vi "trapezoidal.vi"(5 "offset":dbl, 6 "sampling info":cluster{"Fs":dbl, "#s":dbl}={"Fs"=1000.0, "#s"=1000.0} {"Fs" format="%.2p"}, 9 "phase":dbl, 10 "amplitude":dbl, 11 "frequency":i32) -> (2 "signal":waveform(dbl)(graph))   [LabVIEW 2019]
uses:
  <vilib>/Analysis/1siggen.llb/Ramp Pattern by Samples.vi
  <vilib>/Analysis/NI_AALBase.lvlib
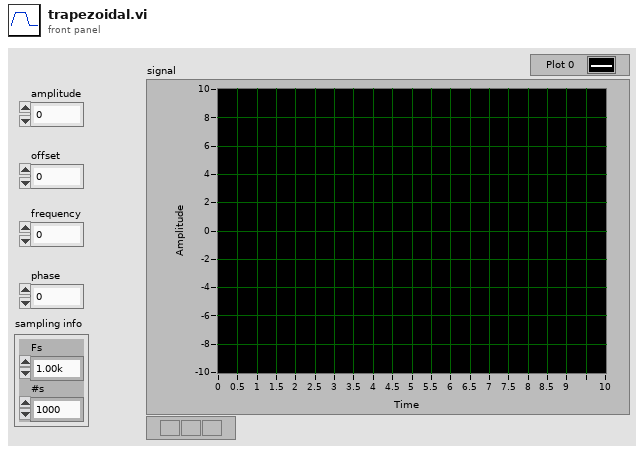
[diagram p1: front panel]
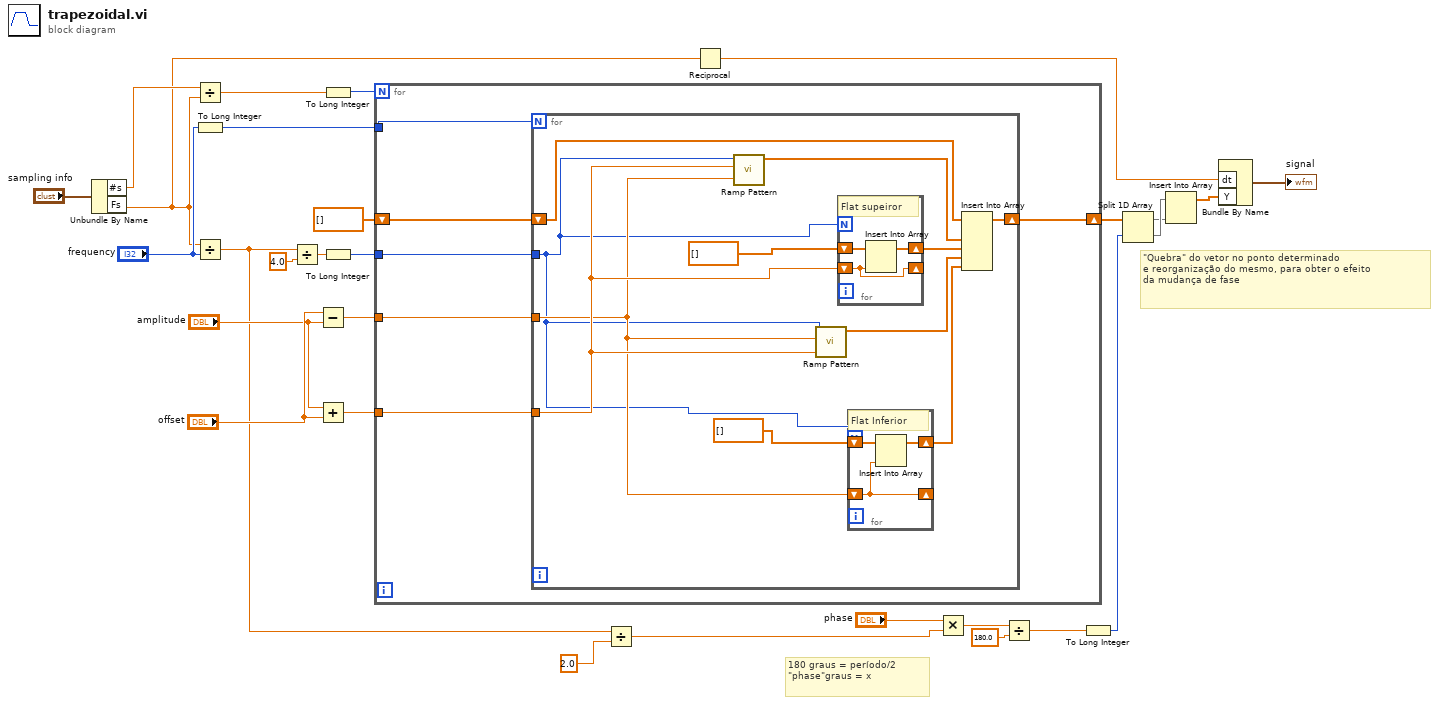
[diagram p0: block diagram]
diagram:
  # "\"Quebra\" do vetor no ponto determinado\ne reorganização do mesmo, para obter o efeito\nda mudança de fase"
  # "180 graus = período/2\n\"phase\"graus = x"
  n1 = Unbundle By Name("sampling info") -> ("#s"=w6:dbl, "Fs"=w5:dbl)
  n2 = Divide(x=w6, y=w5) -> (x/y=w18:dbl)
  n3 = To Long Integer(number="frequency") -> (32bit integer=w20:i32)
  n4 = Divide(x=w5, y="frequency") -> (x/y=w3:dbl)
  n5 = Divide(x=w3, y=4.0) -> (x/y=w23:dbl)
  n6 = Subtract(x="offset", y="amplitude") -> (x-y=w25:dbl)
  n7 = Add(x="amplitude", y="offset") -> (x+y=w28:dbl)
  n8 = To Long Integer(number=w18) -> (32bit integer=w17:i32)
  n9 = To Long Integer(number=w23) -> (32bit integer=w22:i32)
  n10 = for {
    N: w17 -> [_]
    tunnel: w28 -> [w34]
    tunnel: w25 -> [w33]
    tunnel: w22 -> [w32]
    tunnel: w20 -> [w30]
    shift-right: [w35] -> w11
    shift-left: dbl[] [] -> [w31]
    n11 = for {
      N: w30 -> [_]
      tunnel: w34 -> [w46]
      tunnel: w33 -> [w45]
      tunnel: w32 -> [w44]
      shift-right: [w36] -> w35
      shift-left: w31 -> [w43]
      n12 = call-poly <vilib>:"Ramp Pattern.vi"("start"=w45, "end"=w46, "samples"=w44) -> ("Ramp Pattern"=w40:dbl[])  [unwired: 7 in, 1 out]
      n13 = call-poly <vilib>:"Ramp Pattern.vi"("start"=w46, "end"=w45, "samples"=w44) -> ("Ramp Pattern"=w39:dbl[])  [unwired: 7 in, 1 out]
      n14 = for {
        N: w44 -> [_]
        shift-right: [w51] -> w38
        shift-left: dbl[] [] -> [w52]
        shift-right: [w50] -> _
        shift-left: w46 -> [w50]
        # "Flat supeiror"
        n15 = Insert Into Array(array=w52, new element=w50) -> (w51:dbl[])  [unwired: 1 in]
      }
      n16 = for {
        N: w44 -> [_]
        shift-right: [w48] -> w37
        shift-left: dbl[] [] -> [w49]
        shift-right: [w47] -> _
        shift-left: w45 -> [w47]
        # "Flat Inferior"
        n17 = Insert Into Array(array=w49, new element=w47) -> (w48:dbl[])  [unwired: 1 in]
      }
      n18 = Insert Into Array(array=w43, new element #1=w40, new element #2=w38, new element #3=w39, new element #4=w37) -> (w36:dbl[])  [unwired: 1 in]
    }
  }
  n19 = Divide(x=w3, y=2.0) -> (x/y=w1:dbl)
  n20 = Reciprocal(x=w5) -> (1/x=w4:dbl)
  n21 = Multiply(x="phase", y=w1) -> (x*y=w15:dbl)
  n22 = Divide(x=w15, y=180.0) -> (x/y=w16:dbl)
  n23 = To Long Integer(number=w16) -> (32bit integer=w14:i32)
  n24 = Split 1D Array(array=w11, index=w14) -> (first subarray=w9:dbl[], second subarray=w10:dbl[])
  n25 = Insert Into Array(array=w10, new element=w9) -> (w8:dbl[])  [unwired: 1 in]
  n26 = Bundle By Name("dt"=w4, "Y"=w8) -> (→"signal":waveform(dbl))  [unwired: 1 in]
